vi "CRYGet Sound Device Number.vi"(8 "error in (no error)":errorcluster) -> (0 "error out":errorcluster, 2 "Number of Output Devices":i32, 3 "Number of Input Devices":i32)   [LabVIEW 2013]
uses:
  CRYSound.dll
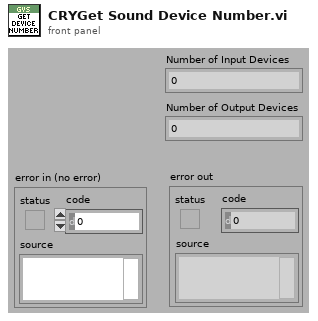
[diagram p1: front panel]
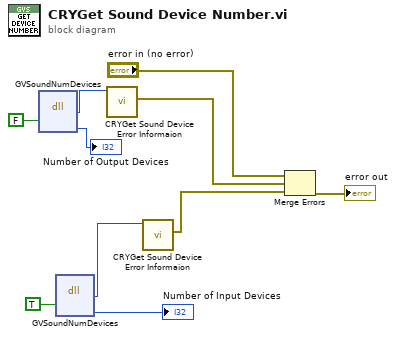
[diagram p0: block diagram]
diagram:
  n1 = dll-call lib="D:/LabView_Project/CRY6181/CRYSound.dll" fn="GVSoundNumDevices"("isInput"=FALSE ("isInput?")) -> ("return type"=w6:i32, "numDevices"=→"Number of Output Devices":i32)  [unwired: 3 in, 4 out]
  n2 = dll-call lib="D:/LabView_Project/CRY6181/CRYSound.dll" fn="GVSoundNumDevices"("isInput"=TRUE ("isInput?")) -> ("return type"=w4:i32, "numDevices"=→"Number of Input Devices":i32)  [unwired: 3 in, 4 out]
  n3 = call "CRYGet Sound Device Error Informaion.vi"("Error Code"=w6) -> ("error out"=w2:errorcluster)  [unwired: 10 out]
  n4 = call "CRYGet Sound Device Error Informaion.vi"("Error Code"=w4) -> ("error out"=w3:errorcluster)  [unwired: 10 out]
  n5 = Merge Errors("error in (no error)", w2, w3) -> (→"error out":errorcluster)
